vi "random-songstructure.vi"(9 "Numeric":i32, 10 "Låst BPM in":i32, 11 "Song structure":T1 {"Outro %" format="%#_13g"; "Solo %" format="%#_13g"; "Bridge %" format="%#_13g"; "Intro %" format="%#_13g"}) -> (2 "String":string, 3 "Song Structure":string[](array[string]))   [LabVIEW 2019]
uses:
  song-structure.ctl
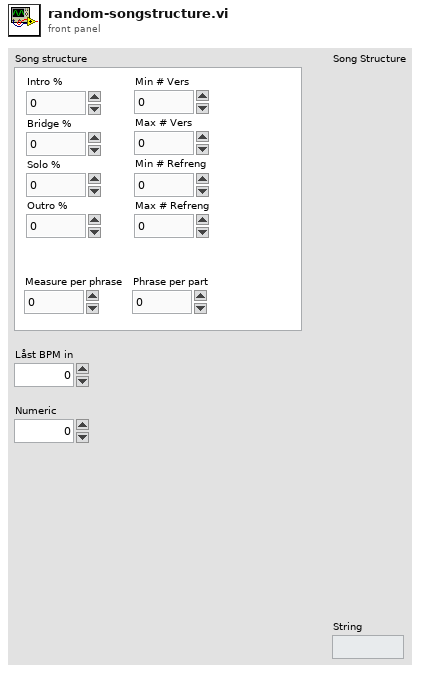
[diagram p1: front panel]
types:
  T1 = typedef "song-structure.ctl" = cluster{"Intro %":dbl, "Bridge %":dbl, "Solo %":dbl, "Outro %":dbl, "Min # Vers":i32, "Max # Vers":i32, "Min # Refreng":i32, "Max # Refreng":i32, "Measure per phrase":i32, "Phrase per part":i32}
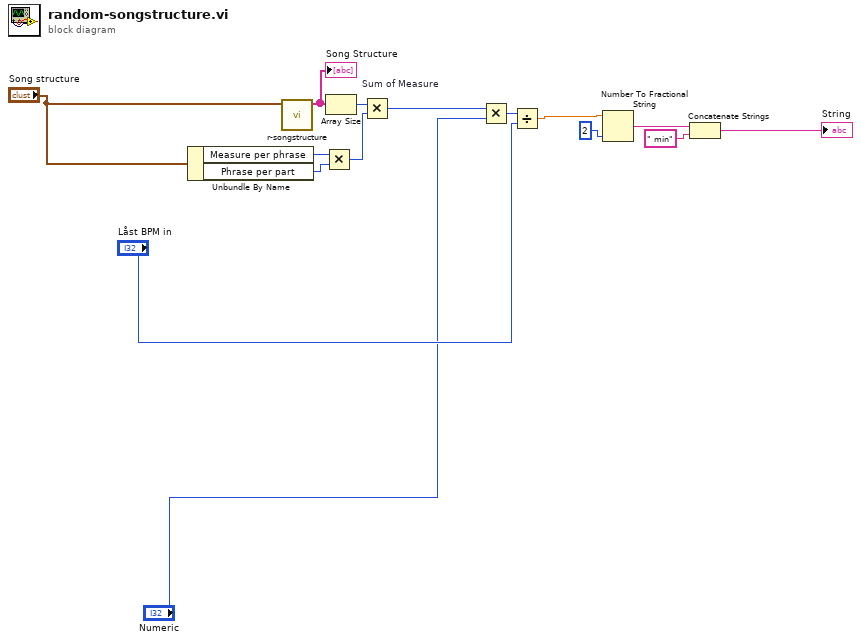
[diagram p0: block diagram]
diagram:
  n1 = Unbundle By Name("Song structure") -> ("Measure per phrase"=w4:i32, "Phrase per part"=w5:i32)
  n2 = call "r-songstructure.vi"("Song structure"="Song structure") -> ("shuffled array"=w2:string[])  [unwired: 10 in]
  "Song Structure" <- w2
  n3 = Multiply(x=w4, y=w5) -> (x*y=w7:i32)
  n4 = Array Size(array=w2) -> (size(s)=w6:i32)
  n5 = Multiply "Sum of Measure"(x=w6, y=w7) -> (x*y=w8:i32)
  n6 = Multiply(x=w8, y="Numeric") -> (x*y=w10:i32)
  n7 = Divide(x=w10, y="Låst BPM in") -> (x/y=w1:dbl)
  n8 = Number To Fractional String(number=w1, precision (6)=i16 2 ("width (-)")) -> (F-format string=w13:string)  [unwired: 2 in]
  n9 = Concatenate Strings(w13, " min" ("string")) -> (→"String":string)
